vi "UI-Cmd-Template.vi"(9 "Data":variant, 10 "Queue":refnum<queue>, 11 "UI State In":T1) -> (0 "error out":errorcluster, 3 "UI State Out":T1)   [LabVIEW 2024, in "CustomActions.lvlib"]
uses:
  CustomActions.lvlib
  UI-State--cluster.ctl
  UI-Refs--cluster.ctl
  UI-Platform--radio.ctl
  UI-ErrorCheckingLevel--radio.ctl
  UI-Cmd--cluster.ctl
  UI-Cmd--enum.ctl
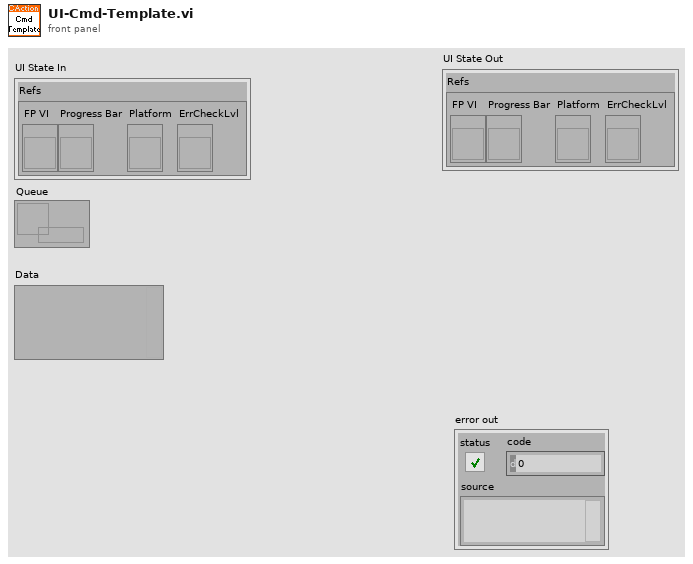
[diagram p1: front panel]
types:
  T1 = typedef "CustomActions.lvlib/UI-State--cluster.ctl" = cluster{"Refs":T2}
  T2 = typedef "CustomActions.lvlib/UI-Refs--cluster.ctl" = cluster{"FP VI":refnum<vi>, "Progress Bar":refnum<vi>, "Platform":refnum<vi>, "ErrCheckLvl":refnum<vi>}
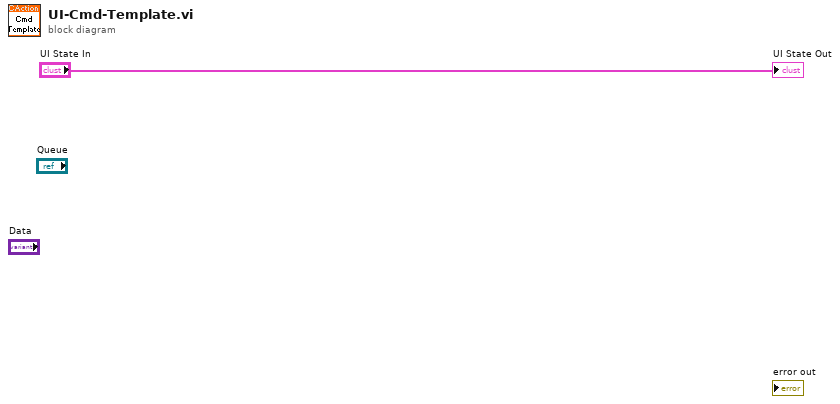
[diagram p0: block diagram]
diagram:
  "UI State Out" <- "UI State In"
